vi "ET3500 - Reference Profile Pt-by-Pt.vi"(5 "Time (sec)":dbl) -> (1 "Ref Temperature":dbl, 2 "data out":dbl[](array[numeric])=[28.24849025386229, 28.23947755526304, 28.19249680418221, 28.285480650091355, 1417.864336646555, 1417.864336646555, 1417.864336646555, 1417.864336646555])   [LabVIEW 2013]
panel:
  # "ni.var.psp://192.168.1.50/RT Library"
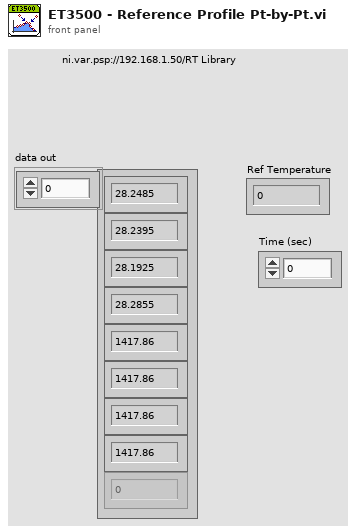
[diagram p1: front panel]
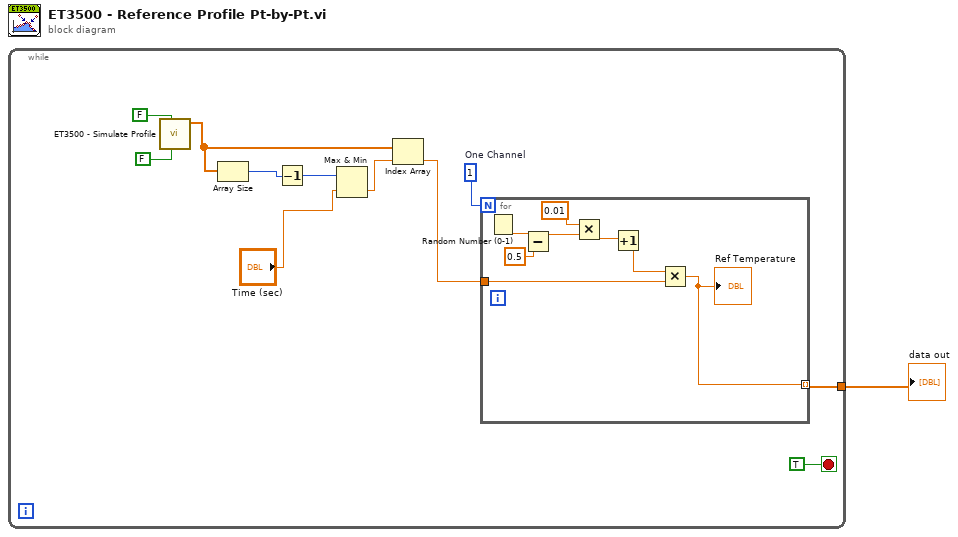
[diagram p0: block diagram]
diagram:
  n1 = while {
    tunnel: [w10] -> w1
    stop <- TRUE stop-if-true
    w4 = 1  # One Channel
    n2 = call "ET3500 - Simulate Profile.vi"("Popup"=FALSE ("subVI"), "Set (T) / Get (F)"=FALSE) -> ("Data"=w7:dbl[])  [unwired: 5 in, 4 out]
    n3 = Array Size(array=w7) -> (size(s)=w6:i32)
    n4 = Decrement(x=w6) -> (x-1=w3:i32)
    n5 = Max & Min(x=w3, y="Time (sec)") -> (min(x,y)=w5:dbl)  [unwired: 1 out]
    n6 = Index Array(array=w7, index=w5) -> (element=w11:dbl)
    n7 = for {
      N: w4 -> [_]
      tunnel: [w14] -> w10 mode=indexing
      tunnel: w11 -> [w15]
      n8 = Random Number (0-1)() -> (number: 0 to 1=w13:dbl)
      n9 = Subtract(x=w13, y=0.5) -> (x-y=w18:dbl)
      n10 = Multiply(x=0.01, y=w18) -> (x*y=w20:dbl)
      n11 = Increment(x=w20) -> (x+1=w16:dbl)
      n12 = Multiply(x=w16, y=w15) -> (x*y=w14:dbl)
      "Ref Temperature" <- w14
    }
  }
  "data out" <- w1
